vi "Manual Triggered Apodization.vi"() -> ()   [LabVIEW 2012]
uses:
  LabVIEW/user.lib/SpectralRadar.llb/Processing Parameter Int Selection.ctl
  LabVIEW/user.lib/SpectralRadar.llb/Probe Parameter Int Selection.ctl
  LabVIEW/user.lib/SpectralRadar.llb/Calibration Selection.ctl
  LabVIEW/user.lib/SpectralRadar.llb/set Spectrum Output.vi
  LabVIEW/user.lib/SpectralRadar.llb/display Data 1D.vi
  LabVIEW/user.lib/SpectralRadar.llb/OCT Device.lvclass
  LabVIEW/user.lib/SpectralRadar.llb/Processing.lvclass
  LabVIEW/user.lib/SpectralRadar.llb/Probe.lvclass
  LabVIEW/user.lib/SpectralRadar.llb/Scan Pattern.lvclass
  LabVIEW/user.lib/SpectralRadar.llb/Raw Data.lvclass
  LabVIEW/user.lib/SpectralRadar.llb/Data.lvclass
panel:
  out "Waveform Graph":dbl[](graph)
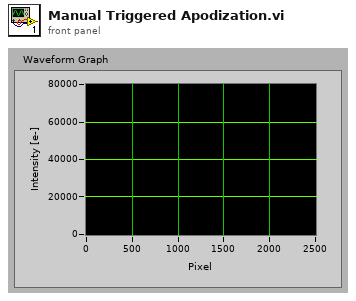
[diagram p1: front panel]
types:
  T1 = typedef "Processing.lvclass/Calibration Selection.ctl" = enum16{"Offset Errors", "Apodization Spectrum", "Apodization Vector", "Dispersion", "Chirp", "Extended Adjust", "Fixed Pattern"}
  T2 = enum16{"Asynchronous Continuous", "Asynchronous Finite", "Synchronous"}
  T3 = typedef "Probe.lvclass/Probe Parameter Int Selection.ctl" = enum16{"Apodization Cycles", "Oversampling", "White Balance Auto", "Oversampling Slow Axis"}
  T4 = typedef "Processing.lvclass/Processing Parameter Int Selection.ctl" = enum32{"Spectrum Averaging", "A-Scan Averaging", "B-Scan Averaging", "Zero Padding", "Number of Threads", "Fourier Averaging"}
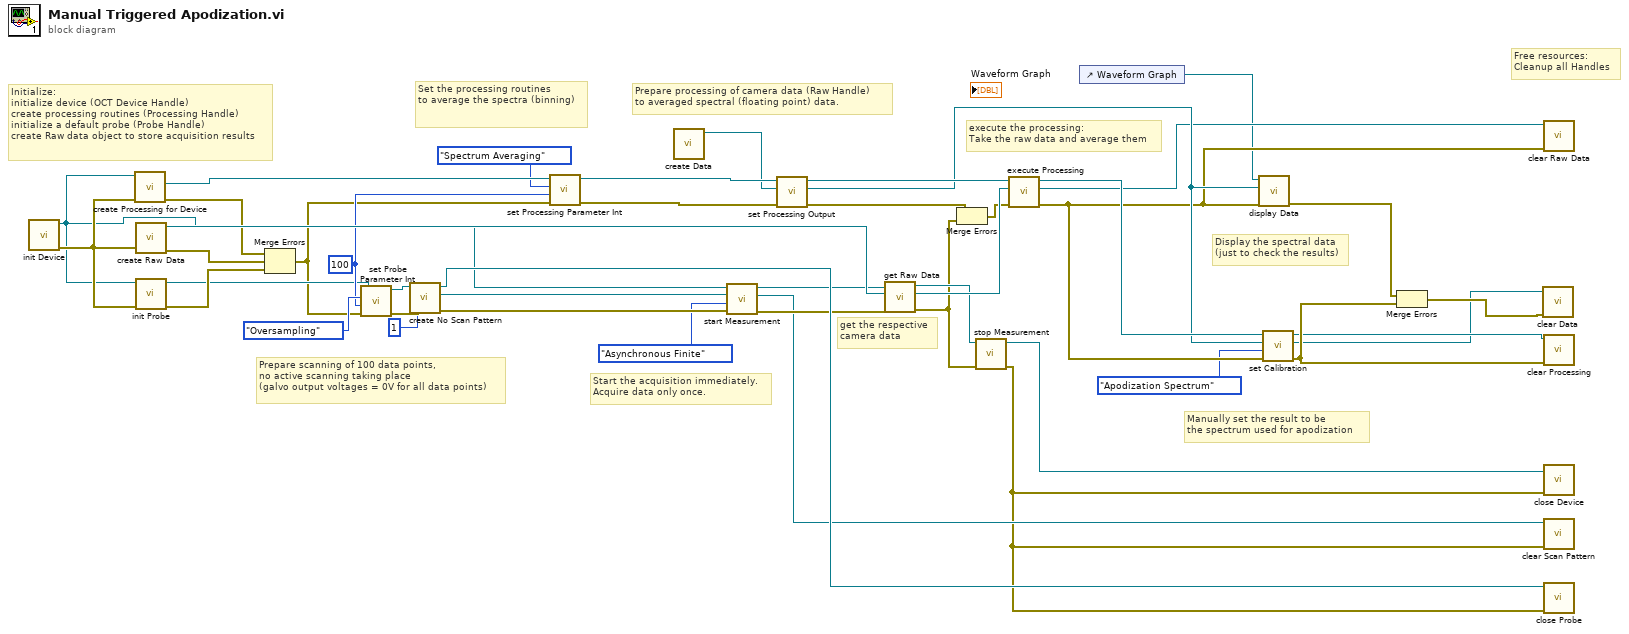
[diagram p0: block diagram]
diagram:
  w29 = 100 ("AScans")
  # "Free resources:\nCleanup all Handles"
  # "Manually set the result to be \nthe spectrum used for apodization"
  # "Display the spectral data\n(just to check the results)"
  # "execute the processing:\nTake the raw data and average them"
  # "get the respective \ncamera data"
  # "Prepare processing of camera data (Raw Handle)\nto averaged spectral (floating point) data."
  # "Start the acquisition immediately.\nAcquire data only once."
  # "Set the processing routines \nto average the spectra (binning)"
  # "Prepare scanning of 100 data points,\nno active scanning taking place \n(galvo output voltages = 0V for all data points)"
  # "Initialize:\ninitialize device (OCT Device Handle)\ncreate processing routines (Processing Handle)\ninitialize a default probe (Probe Handle)\ncreate Raw data object to store acquisition results"
  n1 = call "init Device.vi"() -> ("error out"=w44:errorcluster, "OCTDevice"=w4:refnum<class "OCT Device.lvclass">)  [unwired: 6 in]
  n2 = call "create Processing for Device.vi"("error in (no error)"=w44, "OCTDevice"=w4) -> ("error out"=w41:errorcluster, "Processing"=w43:refnum<class "Processing.lvclass">)  [unwired: 3 in, 1 out]
  n3 = call "create Raw Data.vi"("error in (no error)"=w44) -> ("error out"=w40:errorcluster, "Raw Data"=w42:refnum<class "Raw Data.lvclass">)  [unwired: 5 in]
  n4 = call "init Probe.vi"("error in (no error)"=w44, "OCT Device"=w4) -> ("error out"=w30:errorcluster, "GalvoControl"=w28:refnum<class "Probe.lvclass">)  [unwired: 4 in]
  n5 = Merge Errors(w41, w40, w30) -> (w8:errorcluster)
  n6 = call "set Probe Parameter Int.vi"("error in (no error)"=w8, "Value"=w29, "Probe Parameter Int"=Probe_Parameter_Int_Selection."Oversampling", "GalvoControl"=w28) -> ("error out"=w32:errorcluster, "GalvoControl"=w31:refnum<class "Probe.lvclass">)  [unwired: 2 in]
  n7 = call "create No Scan Pattern.vi"("error in (no error)"=w32, "AScans"=1, "Probe"=w31) -> ("error out"=w39:errorcluster, "Scan Pattern"=w38:refnum<class "Scan Pattern.lvclass">, "Probe"=w34:refnum<class "Probe.lvclass">)  [unwired: 2 in]
  n8 = call "set Processing Parameter Int.vi"("error in (no error)"=w8, "Value"=w29, "Processing Paramter Int Selection"=Processing_Parameter_Int_Selection."Spectrum Averaging", "Processing in"=w43) -> ("error out"=w35:errorcluster, "Processing out"=w37:refnum<class "Processing.lvclass">)  [unwired: 2 in]
  n9 = call "create Data.vi"() -> ("Data"=w3:refnum<class "Data.lvclass">)  [unwired: 6 in, 1 out]
  n10 = call "start Measurement.vi"("error in (no error)"=w39, "Acquisition Type"=T2."Asynchronous Finite", "Scan Pattern"=w38, "OCTDevice"=w4) -> ("error out"=w25:errorcluster, "Scan Pattern"=w14:refnum<class "Scan Pattern.lvclass">, "OCTDevice"=w26:refnum<class "OCT Device.lvclass">)  [unwired: 1 in]
  n11 = call-poly "set Processing Output.vi"("error in (no error)"=w35, "Data"=w3, "Processing"=w37) -> ("error out"=w11:errorcluster, "Data"=w21:refnum<class "Data.lvclass">, "Processing"=w24:refnum<class "Processing.lvclass">)  [unwired: 2 in]
  n12 = call "get Raw Data.vi"("error in (no error)"=w25, "RawData in"=w42, "OCTDevice in"=w26) -> ("error out"=w10:errorcluster, "RawData out"=w23:refnum<class "Raw Data.lvclass">, "OCTDevice out"=w15:refnum<class "OCT Device.lvclass">)  [unwired: 2 in]
  n13 = Merge Errors(w11, w10) -> (w9:errorcluster)
  n14 = call "stop Measurement.vi"("error in (no error)"=w10, "OCTDevice"=w15) -> ("error out"=w12:errorcluster, "OCTDevice"=w13:refnum<class "OCT Device.lvclass">)  [unwired: 4 in]
  n15 = call "execute Processing.vi"("error in (no error)"=w9, "Raw Data"=w23, "Processing"=w24) -> ("error out"=w18:errorcluster, "Raw Data"=w20:refnum<class "Raw Data.lvclass">, "Processing"=w22:refnum<class "Processing.lvclass">)  [unwired: 2 in]
  n16 = control-ref of="Waveform Graph"() -> (w6:refnum<vi>)
  n17 = call-poly "display Data.vi"("error in (no error)"=w18, "Data in"=w21, "WFGraph Refnum"=w6) -> ("error out"=w19:errorcluster)  [unwired: 2 in, 2 out]
  n18 = call "set Calibration.vi"("error in (no error)"=w18, "Calibration Data"=Calibration_Selection."Apodization Spectrum", "Data"=w21, "Processing"=w22) -> ("error out"=w17:errorcluster, "Data"=w1:refnum<class "Data.lvclass">, "Processing"=w16:refnum<class "Processing.lvclass">)  [unwired: 1 in]
  n19 = Merge Errors(w19, w17) -> (w2:errorcluster)
  n20 = call "clear Data.vi"("error in (no error)"=w2, "Data"=w1) -> ()  [unwired: 5 in, 1 out]
  n21 = call "clear Raw Data.vi"("error in (no error)"=w18, "Raw Data"=w20) -> ()  [unwired: 5 in, 1 out]
  n22 = call "clear Processing.vi"("error in (no error)"=w17, "Processing"=w16) -> ()  [unwired: 5 in, 1 out]
  n23 = call "close Device.vi"("error in (no error)"=w12, "OCTDevice"=w13) -> ()  [unwired: 5 in, 1 out]
  n24 = call "clear Scan Pattern.vi"("error in (no error)"=w12, "Scan Pattern in"=w14) -> ()  [unwired: 5 in, 1 out]
  n25 = call "close Probe.vi"("error in (no error)"=w12, "GalvoControl"=w34) -> ()  [unwired: 5 in, 1 out]
